vi "Global rapporto trasfo.vi"() -> ()   [LabVIEW 2019]
panel:
  in  "Rapporto trasfo":dbl
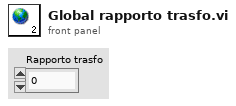
[diagram p1: front panel]
diagram:
